vi "File_FGV_실습.vi"   [LabVIEW 2020]
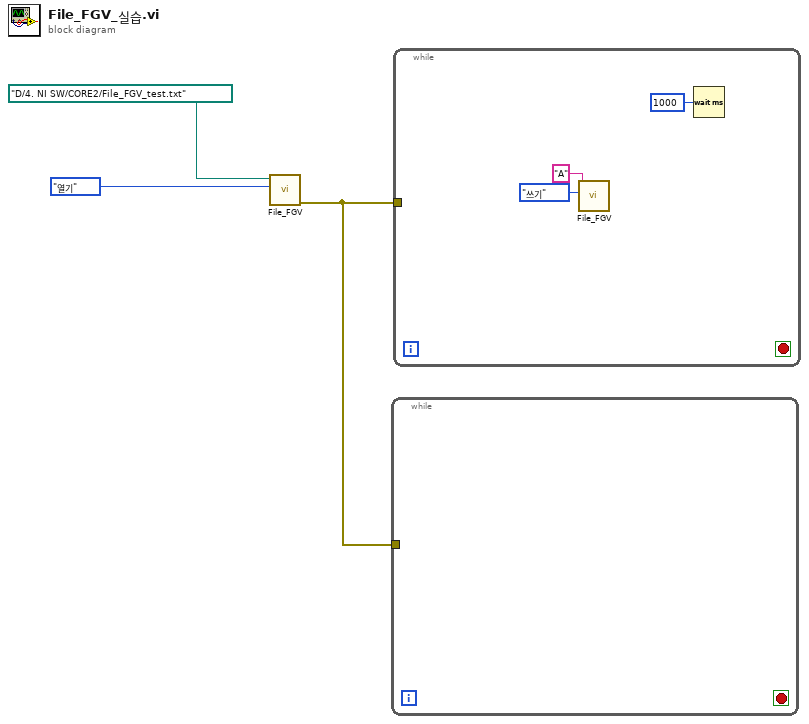
[diagram p0: block diagram]
diagram:
  n1 = call "File_FGV.vi"("열거형"=enum16{"열기", "쓰기", "읽기", "닫기"}."열기", "파일 경로(대화 상자 사용)"=path "D:/4. NI SW/CORE2/File_FGV_test.txt") -> ("에러 출력"=w1:errorcluster)  [unwired: 8 in, 1 out]
  n2 = while {
    tunnel: w1 -> [_]
    stop <- _ stop-if-true
  }
  n3 = while {
    tunnel: w1 -> [_]
    stop <- _ stop-if-true
    n4 = call "File_FGV.vi"("텍스트"="A", "열거형"=enum16{"열기", "쓰기", "읽기", "닫기"}."쓰기") -> ()  [unwired: 8 in, 2 out]
    n5 = Wait (ms)(milliseconds to wait=u32 1000 ("대기 시간 (ms)")) -> ()  [unwired: 1 out]
  }
